vi "RSZVB Get Calibration Data Ports.vi"(8 "error in (no error)":errorcluster {"code" format="%.0x"}, 9 "Calibration (1)":i32=1, 10 "Channel (1)":i32=1, 11 "VISA session":refnum<visa-resource-name>) -> (0 "error out":errorcluster {"code" format="%.0x"}, 2 "Calibration Ports":i32[](array[numeric]), 3 "dup VISA session":refnum<visa-resource-name>)   [LabVIEW 2011]
doc: "This VI queries the calibrated ports.\n\nRemote-control command(s):\n[SENSe<Ch>:]CORRection:DATA:PARameter<Cal>? PORT"
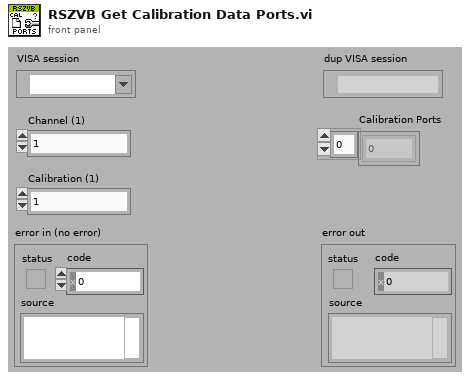
[diagram p1: front panel]
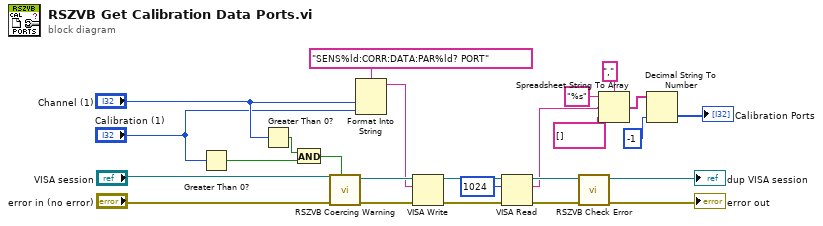
[diagram p0: block diagram]
diagram:
  n1 = Greater Than 0?(x="Calibration (1)") -> (x > 0?=w14:bool)
  n2 = Greater Than 0?(x="Channel (1)") -> (x > 0?=w15:bool)
  n3 = And(x=w15, y=w14) -> (x .and. y?=w16:bool)
  n4 = call "RSZVB Coercing Warning.vi"("In Range?"=w16, "error in (no error)"="error in (no error)", "VISA session"="VISA session") -> ("error out"=w19:errorcluster, "dup VISA session"=w20:refnum<visa-resource-name>)  [unwired: 7 in]
  n5 = Format Into String(format string="SENS%ld:CORR:DATA:PAR%ld? PORT", "Channel (1)", "Calibration (1)") -> (resulting string=w17:string)  [unwired: 2 in, 1 out]
  n6 = VISA Write(VISA resource name=w20, write buffer=w17, error in (no error)=w19) -> (VISA resource name out=w24:refnum<visa-resource-name>, error out=w25:errorcluster)  [unwired: 1 out]
  n7 = VISA Read(VISA resource name=w24, byte count=u32 1024, error in (no error)=w25) -> (VISA resource name out=w21:refnum<visa-resource-name>, read buffer=w5:string, error out=w22:errorcluster)  [unwired: 1 out]
  n8 = call "RSZVB Check Error.vi"("error in (no error)"=w22, "VISA session"=w21) -> ("error out"=→"error out":errorcluster, "dup VISA session"=→"dup VISA session":refnum<visa-resource-name>)  [unwired: 8 in]
  n9 = Spreadsheet String To Array(delimiter (Tab)=",", format string="%s", spreadsheet string=w5, array type (2D Dbl)=string[] []) -> (array=w3:string[])
  n10 = Decimal String To Number(string=w3, default (0L)=-1 ("default (0 I32)")) -> (number=→"Calibration Ports":i32[])  [unwired: 1 in, 1 out]
